vi "Get Header Image.vi"() -> (3 "new picture":picture)   [LabVIEW 2015, in "LVJSON.lvlib" / "Set Object Parameters.xnode"]
uses:
  Set Object Parameters.xnode
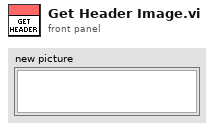
[diagram p1: front panel]
types:
  T1 = typedef "imagedata.ctl" = cluster{"image type":i32, "image depth":i32, "image":u8[], "mask":u8[], "colors":u32[], "Rectangle":cluster{"left":i16, "top":i16, "right":i16, "bottom":i16}}
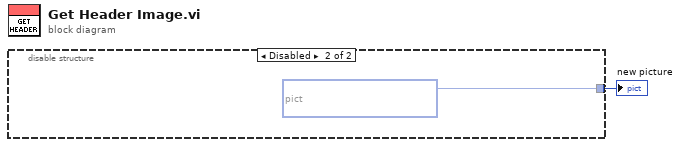
[diagram p0: block diagram]
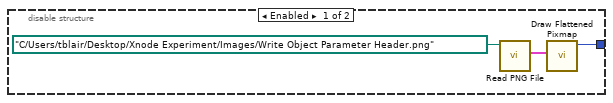
[diagram p2: hidden frame]
diagram:
  n1 = disable-structure shown="Disabled" {
    disable-tunnel: [w2 picture bytes[15070] ("new picture")] -> w1
    frame Enabled {
      n2 = call <vilib>:"Read PNG File.vi"("path to PNG file"=path "C:/Users/tblair/Desktop/Xnode Experiment/Images/Write Object Parameter Header.png") -> ("image data"=w3:T1)  [unwired: 8 in, 2 out]
      n3 = call <vilib>:"Draw Flattened Pixmap.vi"("image data"=w3) -> ("new picture"=w2:picture)  [unwired: 8 in]
    }
    frame Disabled {
    }
  }
  "new picture" <- w1
